vi "PhidgetEnableLogging.vi"(8 "error in":errorcluster, 10 "File Path":path, 11 "LogLevel":i32(ring)=4 items=["CRITICAL"=1, "ERROR"=2, "WARNING"=3, "INFO"=4, "DEBUG"=5, "VERBOSE"=6]) -> (0 "error out":errorcluster)   [LabVIEW 2012, in "Phidget Common.lvlib"]
doc: "Enables logging within the Phidget library."
uses:
  <instrlib>/Phidgets/Phidget Common/Phidget Common.lvlib
  phidget22.dll
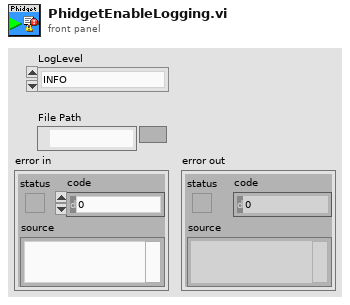
[diagram p1: front panel]
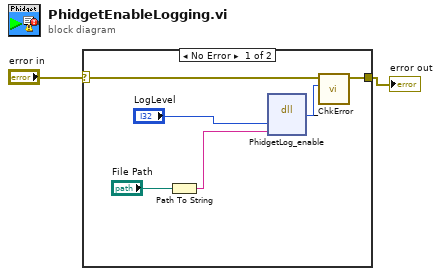
[diagram p0: block diagram]
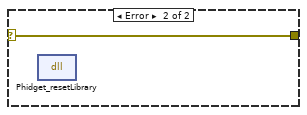
[diagram p2: hidden frame]
diagram:
  n1 = case shown="No Error" "error in" {
    selector: "error in" -> [w8 w9]
    tunnel: [w6 w9] -> w1
    frame No Error {
      n2 = Path To String(path="File Path") -> (string=w3:string)
      n3 = dll-call lib="phidget22.dll" fn="PhidgetLog_enable"("LogLevel"="LogLevel", "Destination"=w3) -> ("return type"=w7:i32)  [unwired: 5 in, 2 out]
      n4 = call <instrlib>:"_ChkError.vi"("Return Code"=w7, "error in (no error)"=w8) -> ("error out"=w6:errorcluster)  [unwired: 9 in]
    }
    frame Error {
      n5 = dll-call lib="phidget22.dll" fn="Phidget_resetLibrary"() -> ()  [unwired: 4 in, 2 out]
    }
  }
  "error out" <- w1
